vi "encodeStream.vi"(8 "error in (no error)":errorcluster, 11 "tBSONDocumentElement in":refnum<class "tBSONDocumentElement.lvclass">) -> (0 "error out":errorcluster, 2 "Byte Array":u8[](array[numeric]), 3 "tBSONDocumentElement out":refnum<class "tBSONDocumentElement.lvclass">)   [LabVIEW 2013, in "BSON.lvlib" / "tBSONDocumentElement.lvclass"]
uses:
  tBSONDocumentElement.lvclass
  tBSONElement/tBSONElement.lvclass
  getValue.vi
  tBSONDocument/tBSONDocument.lvclass
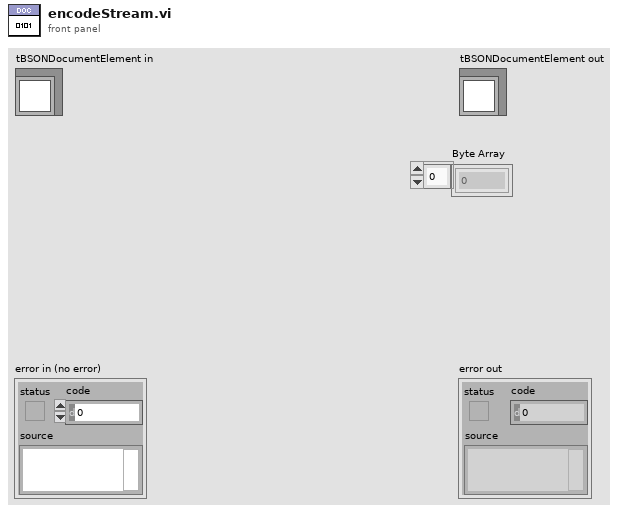
[diagram p1: front panel]
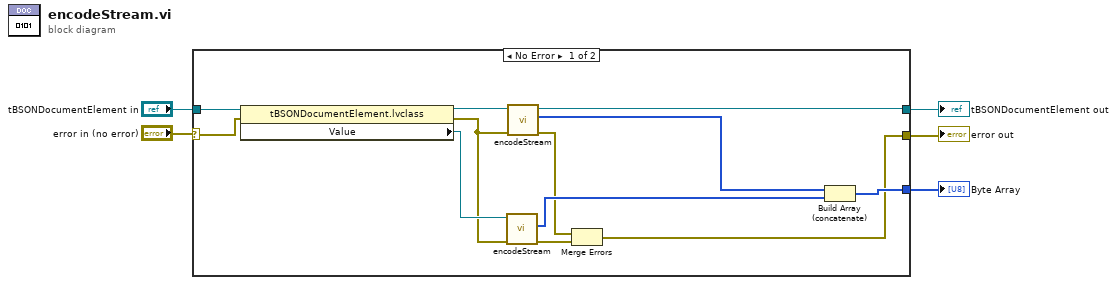
[diagram p0: block diagram]
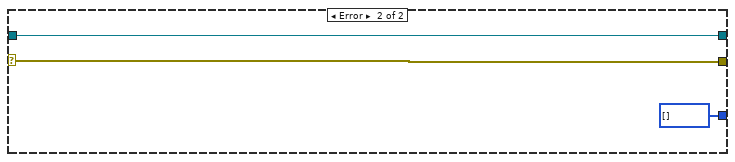
[diagram p2: hidden frame]
diagram:
  n1 = case shown="No Error" "error in (no error)" {
    selector: "error in (no error)" -> [w16 w19]
    tunnel: "tBSONDocumentElement in" -> [w17 w20]
    tunnel: [w9 w20] -> w3
    tunnel: [w11 w19] -> w2
    tunnel: [w12 u8[] []] -> w1
    frame No Error {
      n2 = property class="tBSONDocumentElement.lvclass"(reference=w17, error in=w16) -> (reference out=w10:refnum<class "tBSONDocumentElement.lvclass">, error out=w7:errorcluster, "Value"=w15:refnum<class "tBSONDocument.lvclass">)
      n3 = call "encodeStream.vi"("error in (no error)"=w7, "tBSONDocument in"=w15) -> ("error out"=w13:errorcluster, "Byte Data"=w14:u8[])  [unwired: 7 in, 1 out]
      n4 = call-parent "encodeStream.vi"("error in (no error)"=w7, "tBSONElement in"=w10) -> ("error out"=w8:errorcluster, "Byte Array"=w6:u8[], "tBSONElement out"=w9:refnum<class "tBSONDocumentElement.lvclass">)  [unwired: 7 in]
      n5 = Merge Errors(w8, w13) -> (w11:errorcluster)
      n6 = Build Array (concatenate)(w6, w14) -> (w12:u8[])
    }
    frame Error {
    }
  }
  "error out" <- w2
  "tBSONDocumentElement out" <- w3
  "Byte Array" <- w1
